vi "LabviewDAQTesting.vi"() -> ()   [LabVIEW 2016]
uses:
  <vilib>/Waveform/WDTFileIO.llb/Export Waveform To Spreadsheet File.vi
panel:
  in  "path":path
  out "Numeric":dbl
  out "Wfm7":waveform(dbl)(graph)
  in  "EMG Input Device\nProduct Type":string="USB-6009"
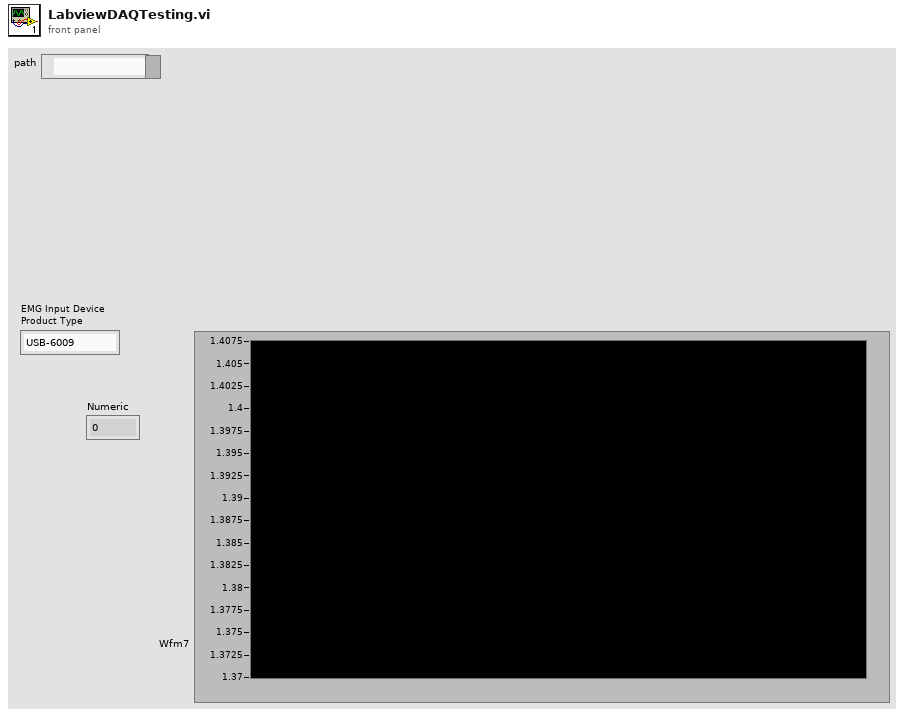
[diagram p1: front panel]
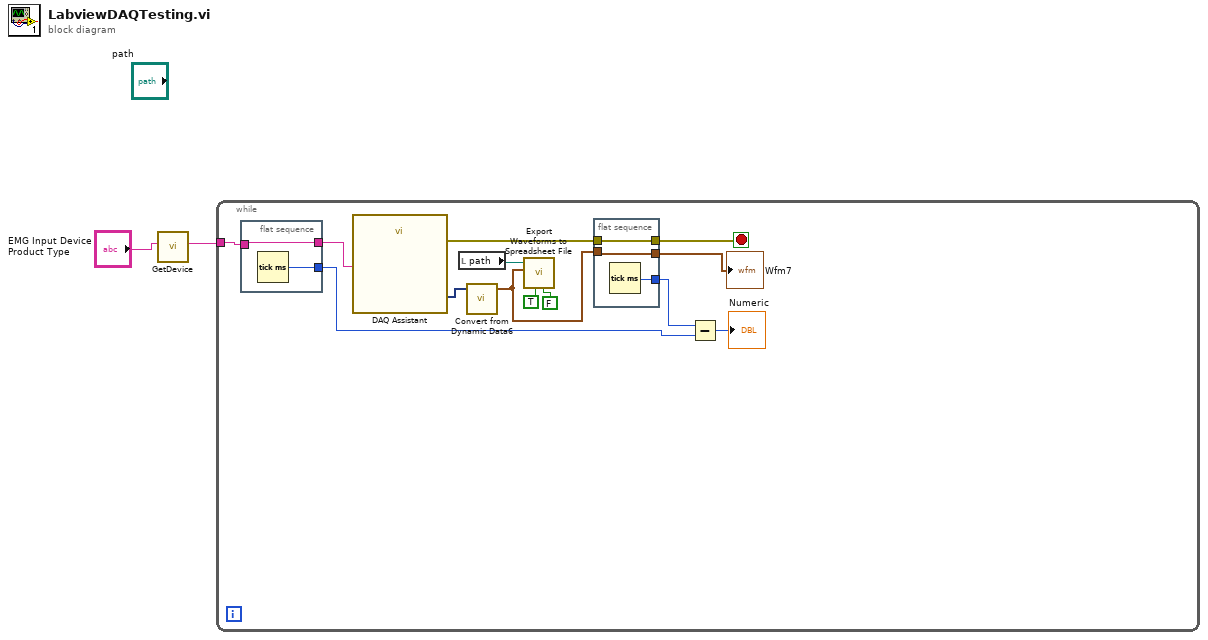
[diagram p0: block diagram]
diagram:
  n1 = call "GetDevice.vi"("EMG Input Device\nProduct Type"="EMG Input Device\nProduct Type") -> ("DAQmx Device Name"=w1:tag)  [unwired: 10 in]
  n2 = while {
    tunnel: w1 -> [w9]
    stop <- w13 stop-if-true
    n3 = flat-sequence {
      tunnel: [w20] -> w15
      tunnel: w9 -> [w20]
      tunnel: [w19] -> w10
      frame #0 {
        n4 = Tick Count (ms)() -> (millisecond timer value=w19:u32)
      }
    }
    n5 = call "DAQ Assistant"("device name"=w15) -> ("data"=w8:dynamicdata, "error out"=w14:errorcluster)  [unwired: 15 in, 2 out]
    n6 = local read "path"() -> (w7:path)
    n7 = call "Convert from Dynamic Data6"("Dynamic Data Type"=w8) -> ("Waveform"=w4:waveform(dbl))  [unwired: 3 in]
    n8 = call-poly <vilib>:"Export Waveforms to Spreadsheet File.vi"("header? (write header:T)"=FALSE, "append to file? (new file:F)"=TRUE, "waveform"=w4, "file path (dialog if empty)"=w7) -> ()  [unwired: 6 in, 2 out]
    n9 = flat-sequence {
      tunnel: [w18] -> w13
      tunnel: w14 -> [w18]
      tunnel: [w17] -> w12
      tunnel: w4 -> [w16]
      tunnel: [w16] -> w3
      frame #0 {
        n10 = Tick Count (ms)() -> (millisecond timer value=w17:u32)
      }
    }
    n11 = Subtract(x=w12, y=w10) -> (x-y=→"Numeric":u32)
    "Wfm7" <- w3
  }
